vi "SetReference2.vi"(0 "DeviceType":u32, 1 "DeviceInd":u32, 2 "CANInd":u32, 3 "RefType":T1 items=["REFTYPE_MODE"=0, "REFTYPE_FILTER"=1, "REFTYPE_ACR0"=2, "REFTYPE_AMR0"=6, "REFTYPE_kCANBAUD"=10, "REFTYPE_CANRX_EN"=13, "REFTYPE_UARTBAUD"=14, "REFTYPE_ALL"=15, "REFTYPE_BRS"=16], 4 "pData":u8[](array[numeric]), 5 "error in (no error)":errorcluster caption="错误输入（无错误）") -> (14 "Success":bool, 19 "error out":errorcluster caption="错误输出")   [LabVIEW 2011]
uses:
  VIs/ParamType.ctl
  data/ControlCAN.dll
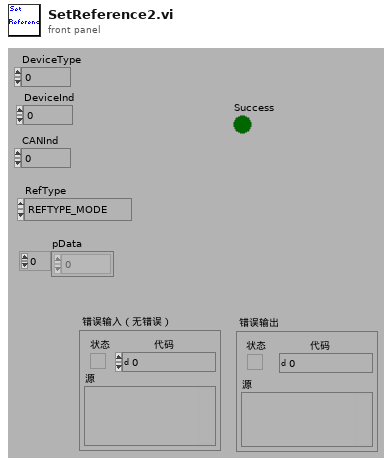
[diagram p1: front panel]
types:
  T1 = typedef "ParamType.ctl" = u32
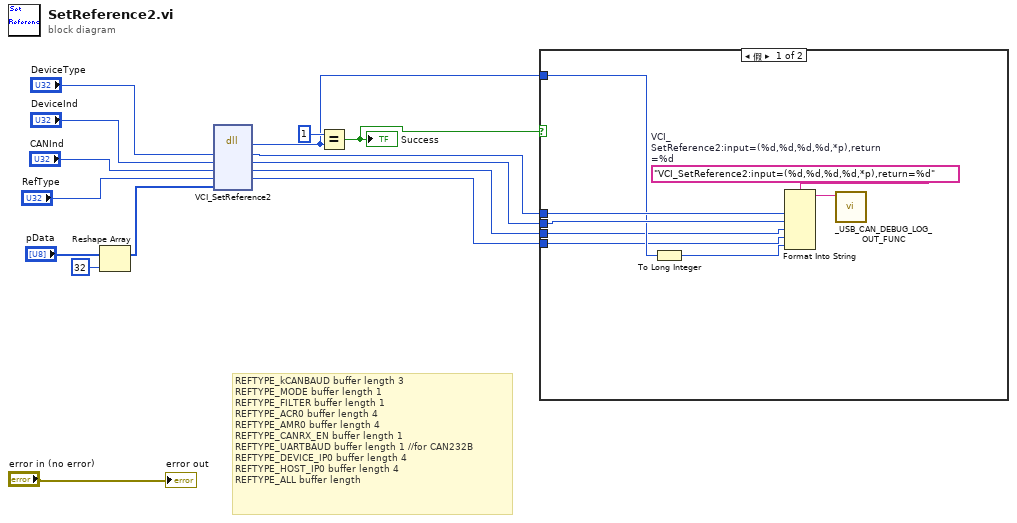
[diagram p0: block diagram]
diagram:
  # "REFTYPE_kCANBAUD buffer length 3\nREFTYPE_MODE buffer length 1\nREFTYPE_FILTER buffer length 1\nREFTYPE_ACR0 buffer length 4\nREFTYPE_AMR0 buffer length 4\nREFTYPE_CANRX_EN buffer length 1\nREFTYPE_UARTBAUD buffer length 1 //for CAN232B\nREFTYPE_DEVICE_IP0 buffer length 4\nREFTYPE_HOST_IP0 buffer length 4\nREFTYPE_ALL buffer length"
  n1 = Reshape Array("pData", 32 ("维数大小")) -> (w9:u8[])
  n2 = dll-call lib="PTH1Mabs ZHost_E工作TnewcodeUSB CAN Tool1.97dataControlCAN.dll" fn="VCI_SetReference2" label="VCI_SetReference"("DeviceType"="DeviceType", "DeviceInd"="DeviceInd", "CANInd"="CANInd", "RefType"="RefType", "pData"=w9) -> ("返回类型"=w5:u32, "DeviceType"=w4:u32, "DeviceInd"=w3:u32, "CANInd"=w2:u32, "RefType"=w1:u32)  [unwired: 4 in, 2 out]
  n3 = Equal?(x=u32 1, y=w5) -> (x = y?=w6:bool)
  "Success" <- w6
  n4 = case shown="假" w6 {
    tunnel: w4 -> [w22 _]
    tunnel: w3 -> [w21 _]
    tunnel: w5 -> [w20 _]
    tunnel: w2 -> [w18 _]
    tunnel: w1 -> [w17 _]
    frame False {
      w19 = "VCI_SetReference2:input=(%d,%d,%d,%d,*p),return=%d"  # VCI_SetReference2:input=(%d,%d,%d,%d,*p),return=%d
      n5 = To Long Integer(number=w20) -> (32bit integer=w16:i32)
      n6 = Format Into String(format string=w19, w22, w21, w18, w17, w16) -> (resulting string=w23:string)  [unwired: 2 in, 1 out]
      n7 = call "_USB_CAN_DEBUG_LOG_OUT_FUNC.vi"("Info"=w23) -> ()  [unwired: 11 in]
    }
    frame True {
    }
  }
  "error out" <- "error in (no error)"
